vi "HAPS_MCU_SerialPort_Readpdet.vi"(5 "Command":string="*IDN?\n", 7 "HAPS_SerialPort_Func":T1, 8 "error in":errorcluster, 10 "Serial Settings":T2={"baud rate"=921600, "data bits"=8, "parity"=enum."None", "stop bits"=10, "flow control"=0} {"flow control" items=["None"=0, "XON/XOFF"=1, "RTS/CTS"=2, "DTR/DSR"=4]; "stop bits" items=["1.0"=10, "1.5"=15, "2.0"=20]; "data bits" min=5 max=8 step=1; "baud rate" items=["75"=75, "110"=110, "134"=134, "150"=150, "300"=300, "600"=600, "1200"=1200, "1800"=1800, "2400"=2400, "4800"=4800, "7200"=7200, "9600"=9600, "14400"=14400, "19200"=19200, "28800"=28800, "38400"=38400, "56000"=56000, "57600"=57600, "115200"=115200, "128000"=128000, "230400"=230400, "921600"=921600]}, 11 "VISA resource name":refnum<visa-resource-name>="COM3") -> (0 "error out":errorcluster, 3 "Command":string, 4 "Time(ms)":dbl)   [LabVIEW 2023, in "HAPS.lvlib"]
uses:
  HAPS_SerialPort.ctl
  <vilib>/Instr/_visa.llb/VISA Configure Serial Port (Instr).vi
  HAPS.lvlib
panel:
  out "r_Data_byte":u32
  in  "delay before read (ms)":u32=5
  out "r_CMD_byte":u32
  out "Data":string
  # "sys_reboot"
  # "ch_ctrl_all\\s0,0,0,0\\r\\n"
  # "set_pd_range\\s0,0,0,9\\r\\n"
  # "get_bfic_temp\\s0,0,0\\r\\n"
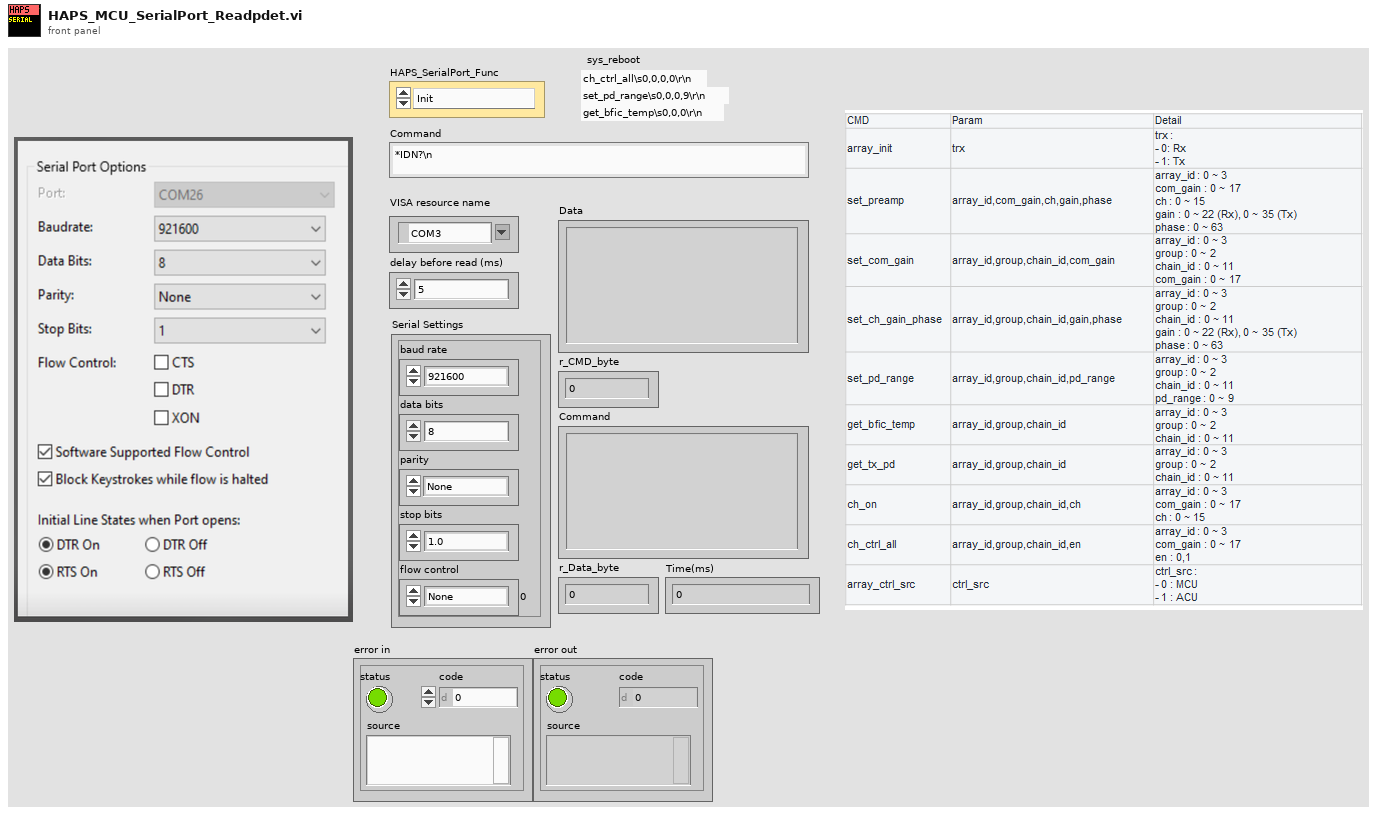
[diagram p1: front panel]
types:
  T1 = typedef "HAPS.lvlib/HAPS_SerialPort.ctl" = enum16{"Init", "Close", "CMD", "Flush"}
  T2 = cluster{"baud rate":u32, "data bits":u16, "parity":enum16{"None", "Odd", "Even", "Mark", "Space"}, "stop bits":u16, "flow control":u16}
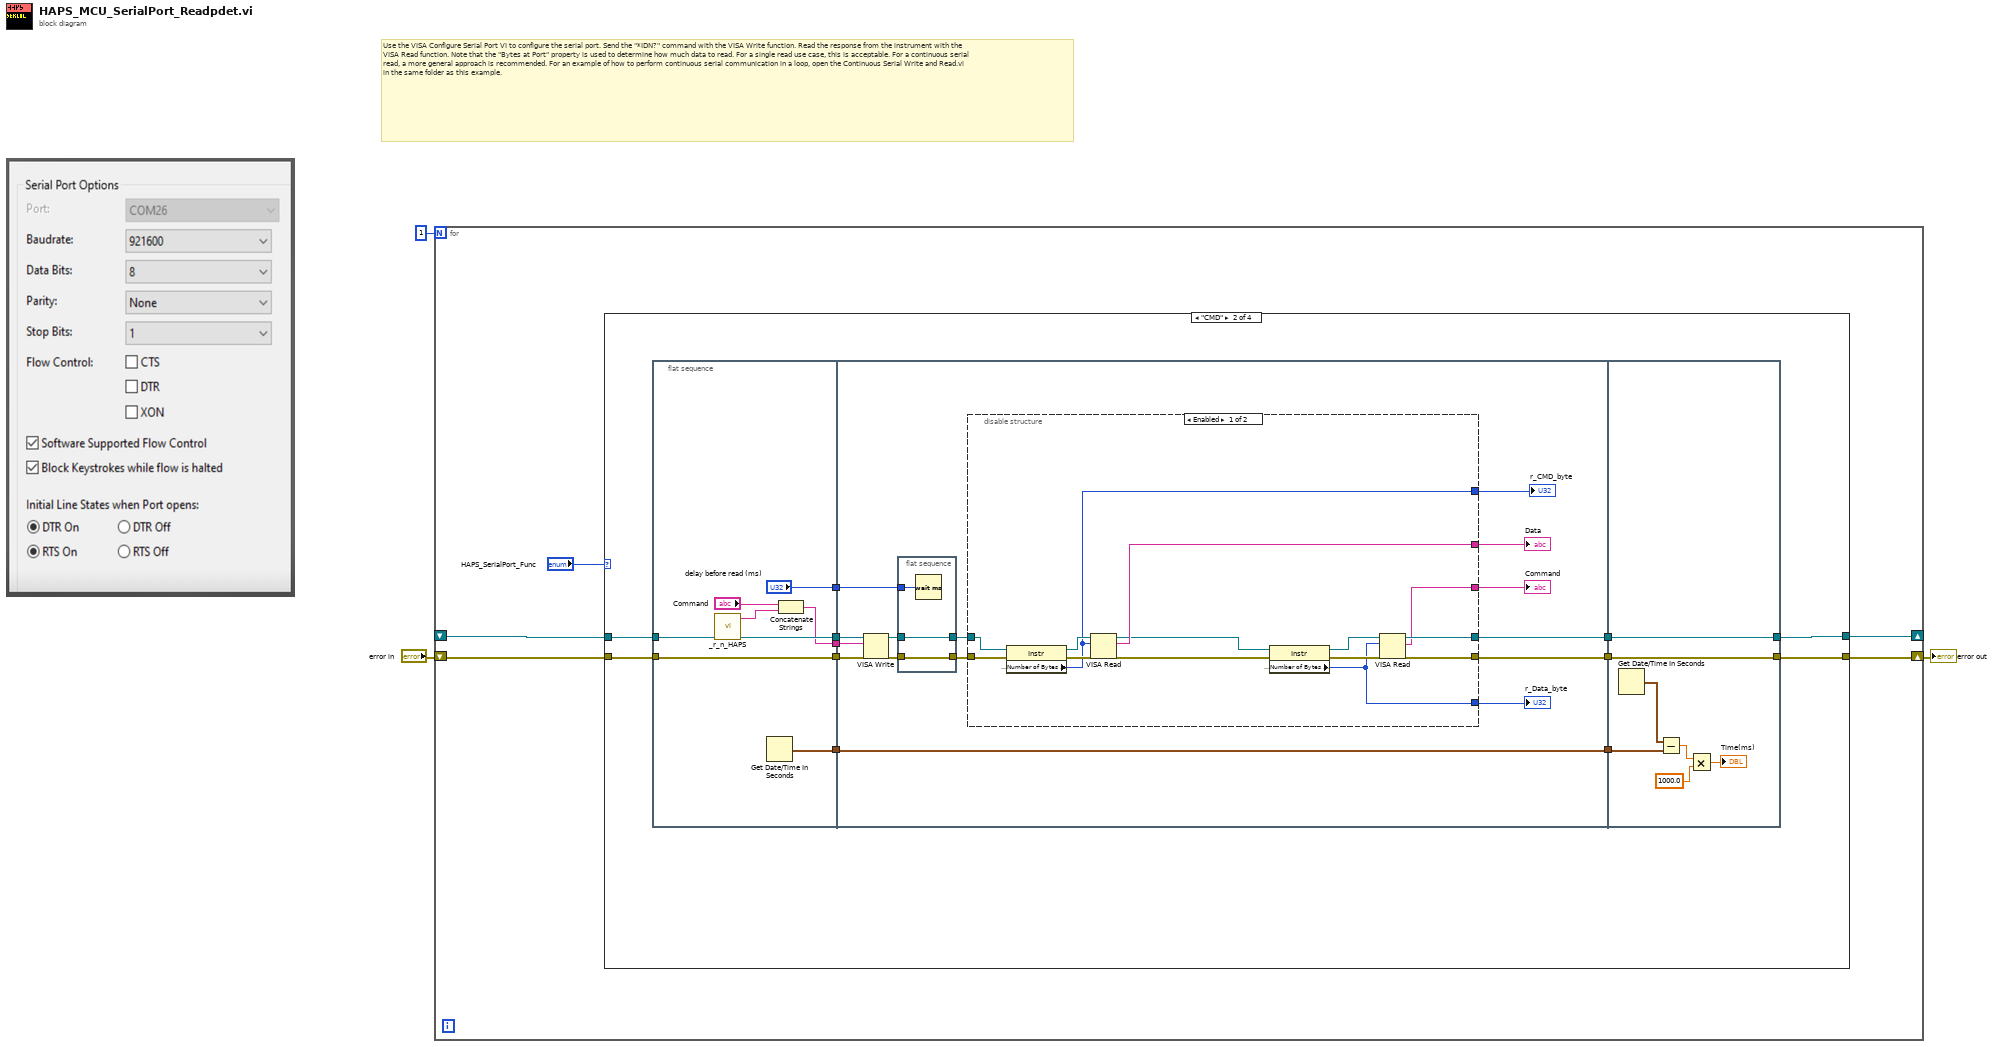
[diagram p0: block diagram]
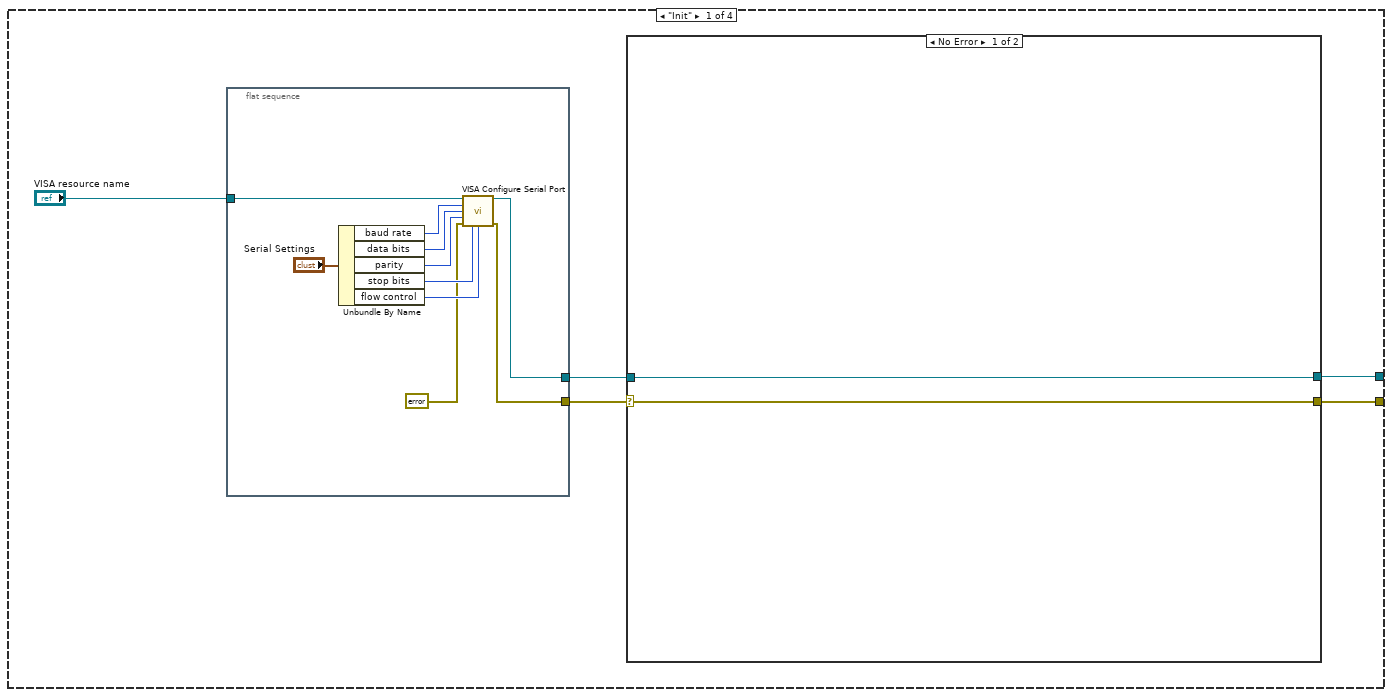
[diagram p2: hidden frame]
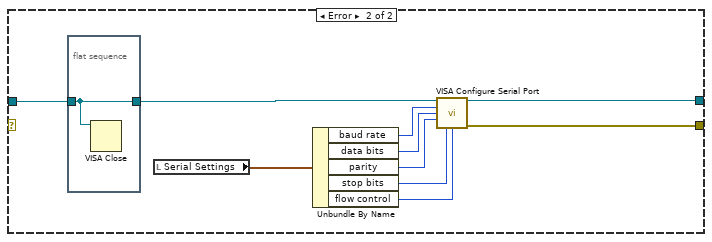
[diagram p3: hidden frame]
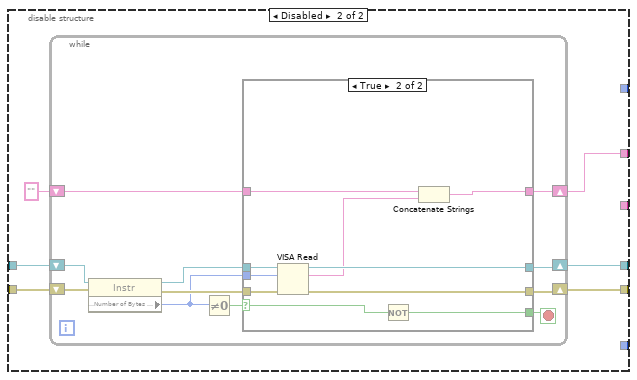
[diagram p4: hidden frame]
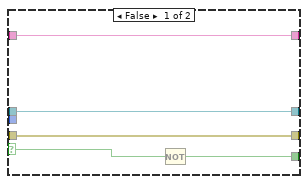
[diagram p5: hidden frame]
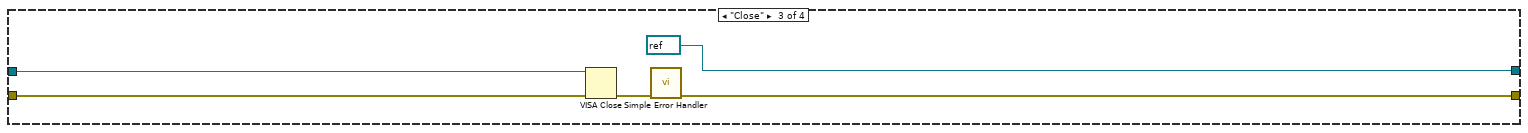
[diagram p6: hidden frame]
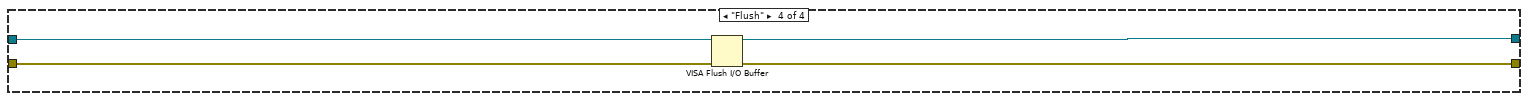
[diagram p7: hidden frame]
diagram:
  # "Use the VISA Configure Serial Port VI to configure the serial port. Send the \"*IDN?\" command with the VISA Write function. Read the response from the instrument with the VISA Read function. Note that the \"Bytes at Port\" property is used to determine how much data to read. For a single read use case, this is acceptable. For a continuous serial read, a more general approach is recommended. For an example of how to perform continuous serial communication in a loop, open the Continuous Serial Write and Read.vi in the same folder as this example."
  n1 = for {
    N: 1 -> [_]
    shift-right: [w6] -> _
    shift-left: _ -> [w7]
    shift-right: [w5] -> w1
    shift-left: "error in" -> [w8]
    n2 = case shown="\"CMD\"" "HAPS_SerialPort_Func" {
      tunnel: w8 -> [_ w40 w130 w135]
      tunnel: w7 -> [_ w39 w128 w133]
      tunnel: [w10 w38 refnum<visa-resource-name> refnum ("VISA resource name out") w132] -> w6
      tunnel: [w12 w37 w129 w134] -> w5
      frame "Init" {
        n3 = flat-sequence {
          tunnel: [w30] -> w13
          tunnel: [w29] -> w11
          tunnel: "VISA resource name" -> [w28]
          frame #0 {
            n4 = Unbundle By Name("Serial Settings") -> ("baud rate"=w32:u32, "data bits"=w33:u16, "parity"=w34:enum16{"None", "Odd", "Even", "Mark", "Space"}, "stop bits"=w35:u16, "flow control"=w36:u16)
            n5 = call-poly "VISA Configure Serial Port"("VISA resource name"=w28, "baud rate (9600)"=w32, "data bits (8)"=w33, "parity (0:none)"=w34, "error in (no error)"=errorcluster {"status"=FALSE, "code"=0, "source"=""}, "stop bits (10: 1 bit)"=w35, "flow control (0:none)"=w36) -> ("VISA resource name out"=w29:refnum<visa-resource-name>, "error out"=w30:errorcluster)  [unwired: 2 in, 5 out]
          }
        }
        n6 = case shown="No Error" w13 {
          selector: w13 -> [w15 _]
          tunnel: [w15 w19] -> w12
          tunnel: w11 -> [w14 w17]
          tunnel: [w14 w18] -> w10
          frame No Error {
          }
          frame Error {
            n7 = flat-sequence {
              tunnel: w17 -> [w26]
              tunnel: [w26] -> w16
              frame #0 {
                n8 = VISA Close(VISA resource name=w26) -> ()  [unwired: 1 in, 1 out]
              }
            }
            n9 = local read "Serial Settings"() -> (w20:T2)
            n10 = Unbundle By Name(w20) -> ("baud rate"=w25:u32, "data bits"=w24:u16, "parity"=w23:enum16{"None", "Odd", "Even", "Mark", "Space"}, "stop bits"=w22:u16, "flow control"=w21:u16)
            n11 = call-poly "VISA Configure Serial Port"("VISA resource name"=w16, "baud rate (9600)"=w25, "data bits (8)"=w24, "parity (0:none)"=w23, "stop bits (10: 1 bit)"=w22, "flow control (0:none)"=w21) -> ("VISA resource name out"=w18:refnum<visa-resource-name>, "error out"=w19:errorcluster)  [unwired: 3 in, 5 out]
          }
        }
      }
      frame "CMD" {
        n12 = flat-sequence {
          tunnel: w39 -> [w54]
          tunnel: w40 -> [w55]
          tunnel: [w55] -> w48
          tunnel: [w54] -> w47
          tunnel: ["delay before read (ms)"] -> w46
          tunnel: [w50] -> w45
          tunnel: [w53] -> w44
          tunnel: w48 -> [w70]
          tunnel: w47 -> [w69]
          tunnel: w46 -> [w66]
          tunnel: w45 -> [w65]
          tunnel: [w60] -> w43
          tunnel: [w59] -> w42
          tunnel: w44 -> [w56]
          tunnel: [w56] -> w41
          tunnel: [w120] -> w38
          tunnel: [w121] -> w37
          tunnel: w43 -> [w121]
          tunnel: w42 -> [w120]
          tunnel: w41 -> [w126]
          frame #0 {
            n13 = call "_r_n_HAPS.vi"() -> ("command"=w49:string)  [unwired: 5 in]
            n14 = Get Date/Time In Seconds() -> (seconds since 1Jan1904=w53:timestamp)
            n15 = Concatenate Strings("Command", w49) -> (w50:string)
          }
          frame #1 {
            n16 = VISA Write(VISA resource name=w69, write buffer=w65, error in (no error)=w70) -> (VISA resource name out=w67:refnum<visa-resource-name>, error out=w68:errorcluster)  [unwired: 1 out]
            n17 = flat-sequence {
              tunnel: w68 -> [w118]
              tunnel: [w118] -> w63
              tunnel: w67 -> [w117]
              tunnel: [w117] -> w62
              tunnel: w66 -> [w119]
              frame #0 {
                n18 = Wait (ms)(milliseconds to wait=w119) -> ()  [unwired: 1 out]
              }
            }
            n19 = disable-structure shown="Enabled" {
              disable-tunnel: [w82 w85] -> w64
              disable-tunnel: w63 -> [w81 w90]
              disable-tunnel: w62 -> [w80 w89]
              disable-tunnel: [w79 _] -> w61
              disable-tunnel: [w78 w86] -> w60
              disable-tunnel: [w77 w87] -> w59
              disable-tunnel: [w72 _] -> w58
              disable-tunnel: [w71 _] -> w57
              frame Enabled {
                n20 = property class="Instr"(reference=w80, error in=w81) -> (reference out=w84:refnum<visa-resource-name>, error out=w83:errorcluster, "Serial Settings:Number of Bytes at Serial Port"=w79:u32)
                n21 = VISA Read(VISA resource name=w84, byte count=w79, error in (no error)=w83) -> (VISA resource name out=w76:refnum<visa-resource-name>, read buffer=w82:string, error out=w75:errorcluster)  [unwired: 1 out]
                n22 = property class="Instr"(reference=w76, error in=w75) -> (reference out=w73:refnum<visa-resource-name>, error out=w74:errorcluster, "Serial Settings:Number of Bytes at Serial Port"=w71:u32)
                n23 = VISA Read(VISA resource name=w73, byte count=w71, error in (no error)=w74) -> (VISA resource name out=w77:refnum<visa-resource-name>, read buffer=w72:string, error out=w78:errorcluster)  [unwired: 1 out]
              }
              frame Disabled {
                n24 = while {
                  shift-right: [w95] -> w86
                  shift-left: w90 -> [w99]
                  shift-right: [w91] -> w87
                  shift-left: w89 -> [w98]
                  shift-right: [w93] -> w85
                  shift-left: "" -> [w94]
                  stop <- w92 stop-if-true
                  n25 = property class="Instr"(reference=w98, error in=w99) -> (reference out=w101:refnum<visa-resource-name>, error out=w100:errorcluster, "Serial Settings:Number of Bytes at Serial Port"=w97:u32)
                  n26 = Not Equal To 0?(x=w97) -> (x != 0?=w96:bool)
                  n27 = case shown="True" w96 {
                    selector: w96 -> [w104 w108]
                    tunnel: w101 -> [w102 w116]
                    tunnel: w100 -> [w106 w115]
                    tunnel: w97 -> [_ w114]
                    tunnel: [w102 w113] -> w91
                    tunnel: [w106 w112] -> w95
                    tunnel: w94 -> [w105 w111]
                    tunnel: [w105 w109] -> w93
                    tunnel: [w103 w107] -> w92
                    frame False {
                      n28 = Not(x=w104) -> (.not. x?=w103:bool)
                    }
                    frame True {
                      n29 = VISA Read(VISA resource name=w116, byte count=w114, error in (no error)=w115) -> (VISA resource name out=w113:refnum<visa-resource-name>, read buffer=w110:string, error out=w112:errorcluster)  [unwired: 1 out]
                      n30 = Not(x=w108) -> (.not. x?=w107:bool)
                      n31 = Concatenate Strings(w111, w110) -> (w109:string)
                    }
                  }
                }
              }
            }
            "Data" <- w64
            "r_CMD_byte" <- w61
            "Command" <- w58
            "r_Data_byte" <- w57
          }
          frame #2 {
            n32 = Get Date/Time In Seconds() -> (seconds since 1Jan1904=w125:timestamp)
            n33 = Subtract(x=w125, y=w126) -> (x-y=w122:dbl)
            n34 = Multiply(x=w122, y=1000.0) -> (x*y=→"Time(ms)":dbl)
          }
        }
      }
      frame "Close" {
        n35 = VISA Close(VISA resource name=w128, error in (no error)=w130) -> (error out=w131:errorcluster)
        n36 = call <vilib>:"Simple Error Handler.vi"("error in (no error)"=w131) -> ("error out"=w129:errorcluster)  [unwired: 1 in, 7 out]
      }
      frame "Flush" {
        n37 = VISA Flush I/O Buffer(VISA resource name=w133, error in (no error)=w135) -> (VISA resource name out=w132:refnum<visa-resource-name>, error out=w134:errorcluster)  [unwired: 1 in]
      }
    }
  }
  "error out" <- w1
